vi "Write Config.vi"(8 "error in (no error)":errorcluster, 10 "Config.lvlibp:Config.lvclass":refnum<class "Config.lvclass">, 11 "Configuration UI in":refnum<class "Configuration UI.lvclass">) -> (0 "error out":errorcluster, 3 "Configuration UI out":refnum<class "Configuration UI.lvclass">)   [LabVIEW 2019, in "Configuration UI.lvlib" / "Configuration UI.lvclass"]
uses:
  Project/Configuration UI.lvclass
  builds/Tools/Config.lvlibp/Config.lvclass
  Project/Configuration UI.lvclass/Configuration UI.ctl
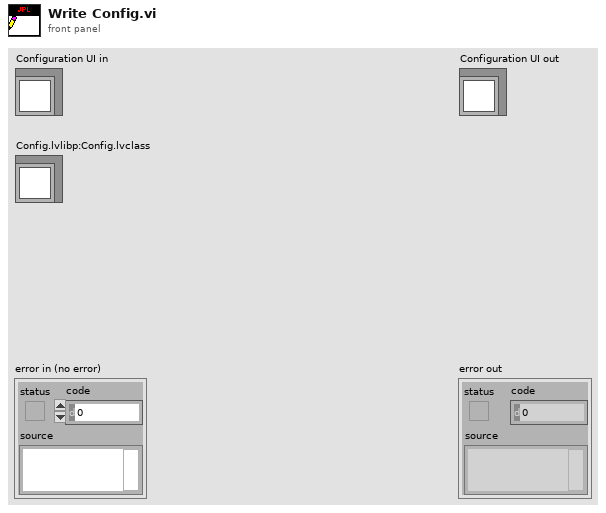
[diagram p1: front panel]
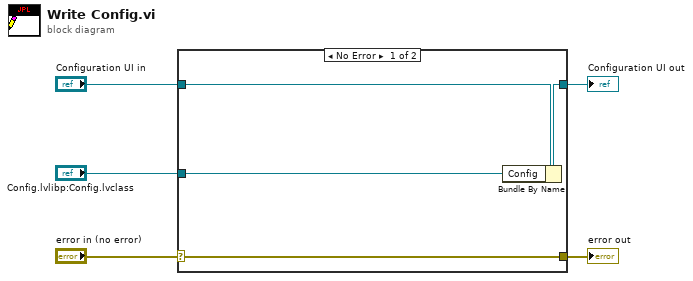
[diagram p0: block diagram]
diagram:
  n1 = case shown="No Error" "error in (no error)" {
    selector: "error in (no error)" -> [w9 w10]
    tunnel: [w9 w10] -> w4
    tunnel: [w7 w11] -> w2
    tunnel: "Configuration UI in" -> [w8 w11]
    tunnel: "Config.lvlibp:Config.lvclass" -> [w6 _]
    frame No Error {
      n2 = Bundle By Name(cluster=w8, "Config"=w6) -> (w7:refnum<class "Configuration UI.lvclass">)
    }
    frame Error {
    }
  }
  "error out" <- w4
  "Configuration UI out" <- w2
